vi "Path to Short Name.vi"(8 "error in":errorcluster, 11 "Path":refnum<class "UTF-8 Path.lvclass">) -> (0 "error out":errorcluster, 3 "LabVIEW Path":path)   [LabVIEW 2020, in "G-Unicode.lvlib"]
doc: "Converts the UTF-8 path to the corresponding 8.3 short name path. Note that the path must exist on disk.\n\nThe short name path is ASCII encoded, and can be used by LabVIEW's standard file I/O functions. This allows accessing unicode paths within LabVIEW.\n\n<b>Windows only.</b> Linux and macOS will return a UTF-8 encoded path."
uses:
  G-Unicode.lvlib
  kernel32.dll
  2ac34a2c-f2f8-4f46-8fc4-84da909d2cd5.vi
  f844562b-b612-4fa1-b092-3cf87b2107aa.vi
  Types/UTF-8 String/UTF-8 String.lvclass
  Types/UTF-8 Path/UTF-8 Path.lvclass
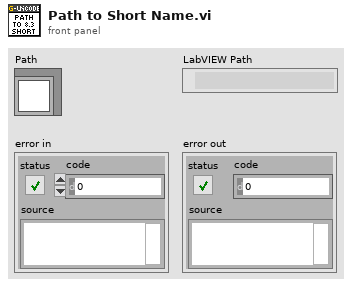
[diagram p1: front panel]
types:
  T1 = typedef "G-Unicode.lvlib/Encoded UTF-8 String.ctl" = string
  T2 = typedef "G-Unicode.lvlib/Encoded UTF-16LE String.ctl" = string
  T3 = typedef "G-Unicode.lvlib/Encoded UTF-8 Path.ctl" = path
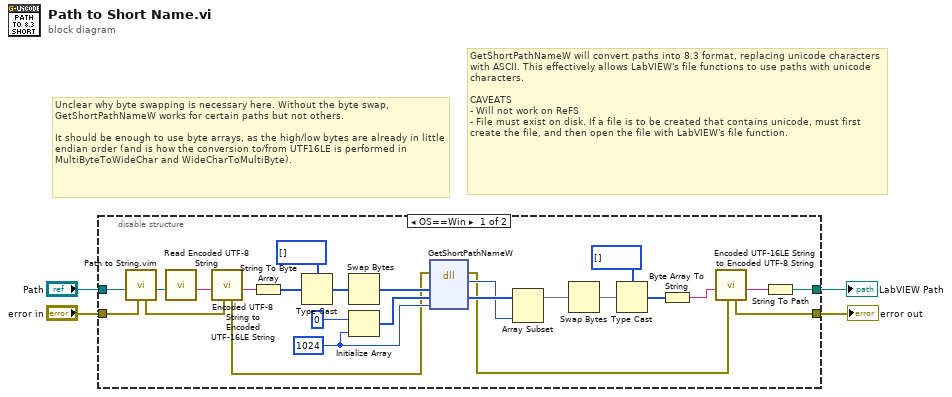
[diagram p0: block diagram]
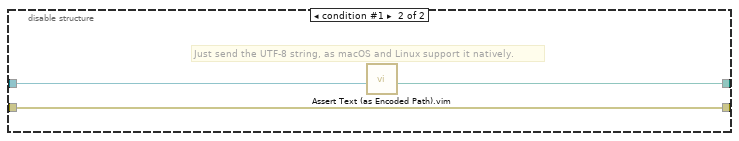
[diagram p2: hidden frame]
diagram:
  # "GetShortPathNameW will convert paths into 8.3 format, replacing unicode characters with ASCII. This effectively allows LabVIEW's file functions to use paths with unicode characters.\n\nCAVEATS\n- Will not work on ReFS\n- File must exist on disk. If a file is to be created that contains unicode, must first create the file, and then open the file with LabVIEW's file function."
  # "Unclear why byte swapping is necessary here. Without the byte swap, GetShortPathNameW works for certain paths but not others.\n\nIt should be enough to use byte arrays, as the high/low bytes are already in little endian order (and is how the conversion to/from UTF16LE is performed in MultiByteToWideChar and WideCharToMultiByte)."
  n1 = disable-structure shown="OS==Win" {
    disable-tunnel: [w12 w30] -> w1
    disable-tunnel: "Path" -> [w11 w31]
    disable-tunnel: "error in" -> [w10 w32]
    disable-tunnel: [w14 w32] -> w2
    frame condition #0 (active) {
      w27 = u32 1024 ("dimension size")
      n2 = call "Path to String.vim"("error in"=w10, "Path"=w11) -> ("String"=w9:refnum<class "UTF-8 String.lvclass">, "error out"=w7:errorcluster)  [unwired: 8 in]
      n3 = call "Read Encoded UTF-8 String.vi"("UTF-8 String"=w9) -> ("Encoded UTF-8 String"=w8:T1)  [unwired: 10 in]
      n4 = call "Encoded UTF-8 String to Encoded UTF-16LE String.vi"("error in"=w7, "Encoded UTF-8 String"=w8) -> ("Encoded UTF-16LE String"=w5:T2, "error out"=w6:errorcluster)  [unwired: 8 in]
      n5 = String To Byte Array(string=w5) -> (unsigned byte array=w20:u8[])
      n6 = Type Cast(type=u16[] [], x=w20) -> (*(type *) &x=w25:u16[])
      n7 = Swap Bytes(anything=w25) -> (byte swapped=w18:u16[])
      n8 = Initialize Array(u16 0 ("element"), w27) -> (w28:u16[])
      n9 = dll-call lib="kernel32.dll" fn="GetShortPathNameW"(error in=w6, "lpszLongPath"=w18, "lpszShortPath"=w28, "cchBuffer"=w27) -> (error out=w15:errorcluster, "return type"=w17:u32, "lpszShortPath"=w24:u16[])  [unwired: 4 in, 1 out]
      n10 = Array Subset(array=w24, length=w17) -> (w19:u16[])  [unwired: 1 in]
      n11 = Swap Bytes(anything=w19) -> (byte swapped=w22:u16[])
      n12 = Type Cast(type=u8[] [], x=w22) -> (*(type *) &x=w16:u8[])
      n13 = Byte Array To String(unsigned byte array=w16) -> (string=w26:string)
      n14 = call "Encoded UTF-16LE String to Encoded UTF-8 String.vi"("error in"=w15, "Encoded UTF-16LE String"=w26) -> ("Encoded UTF-8 String"=w13:T1, "error out"=w14:errorcluster)  [unwired: 8 in]
      n15 = String To Path(string=w13) -> (path=w12:path)
    }
    frame condition #1 {
      # "Just send the UTF-8 string, as macOS and Linux support it natively."
      n16 = call "Assert Text (as Encoded Path).vim"("Text"=w31) -> ("Encoded Path"=w30:T3)  [unwired: 9 in, 1 out]
    }
  }
  "LabVIEW Path" <- w1
  "error out" <- w2
